vi "Set Connection.vi"(8 "error in (no error)":errorcluster, 9 "TCP Stream":refnum<class "TCP Stream.lvclass">, 10 "TCP Connection":refnum<k5>, 11 "TCP Client in":refnum<class "TCP Client.lvclass">) -> (0 "error out":errorcluster, 3 "TCP Client out":refnum<class "TCP Client.lvclass">)   [LabVIEW 2020, in "Stream-TCP.lvlib" / "TCP Client.lvclass"]
uses:
  TCP Client.lvclass
  TCP Stream/TCP Stream.lvclass
  TCP Client.lvclass/TCP Client.ctl
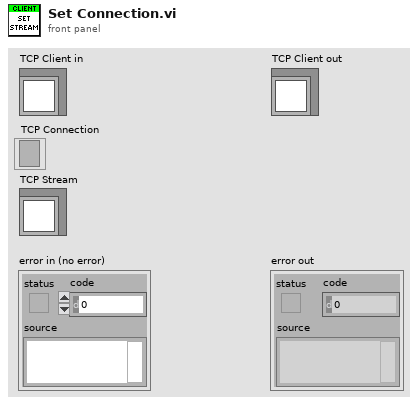
[diagram p1: front panel]
types:
  T1 = typedef "Stream-TCP.lvlib/TCP Client.lvclass/Ref Data.ctl" = cluster{"TCP Connection":refnum<k5>, "TCP Stream":refnum<class "TCP Stream.lvclass">, "State":T2, "Connection Loop":refnum<vi>, "TCP Mode":T3, "Timeout ms":i32, "Server Connection":bool}
  T2 = typedef "Stream-TCP.lvlib/TCP Client.lvclass/Connection State.ctl" = enum16{"Closed", "Idle", "Connecting", "Connected", "Shutdown"}
  T3 = typedef "Stream-TCP.lvlib/TCP Mode.ctl" = enum16{"buffered", "raw"}
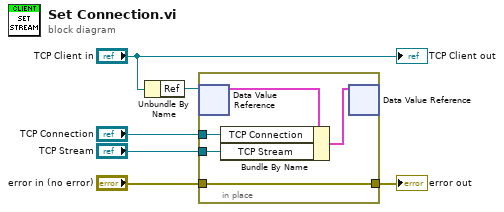
[diagram p0: block diagram]
diagram:
  n1 = Unbundle By Name("TCP Client in") -> ("Ref"=w6:refnum<data-value>)
  n2 = in-place {
    in-place-border: "TCP Connection" -> [w9]
    in-place-border: "TCP Stream" -> [w8]
    in-place-border: "error in (no error)" -> [w7]
    in-place-border: [w7] -> w1
    n3 = in-place-dvr #1(w6) -> (w11:T1)  [unwired: 1 out]
    n4 = Bundle By Name(cluster=w11, "TCP Connection"=w9, "TCP Stream"=w8) -> (w10:T1)
    n5 = in-place-dvr #1(w10) -> ()  [unwired: 2 out]
  }
  "error out" <- w1
  "TCP Client out" <- "TCP Client in"
